vi "appEntry.vi"() -> ()   [LabVIEW 2018]
uses:
  type_sa_visit.ctl
  <vilib>/addons/database/Connection.llb/DB Tools Open Connec (String).vi
  <vilib>/addons/database/Connection.llb/Conn Execute.vi
  <vilib>/addons/database/Recordset.llb/Rec Fetch Recordset Data (R).vi
  <vilib>/addons/database/_DB Variant To Data/Database Variant To Data.xnode
  <vilib>/addons/database/NI_Database_API.lvlib
panel:
  in  "选项卡控件":enum32{"信息查询", "宿舍管理", "公寓管理", "系统管理"}(tab)
  in  "type_stu_apartment_visit":T1
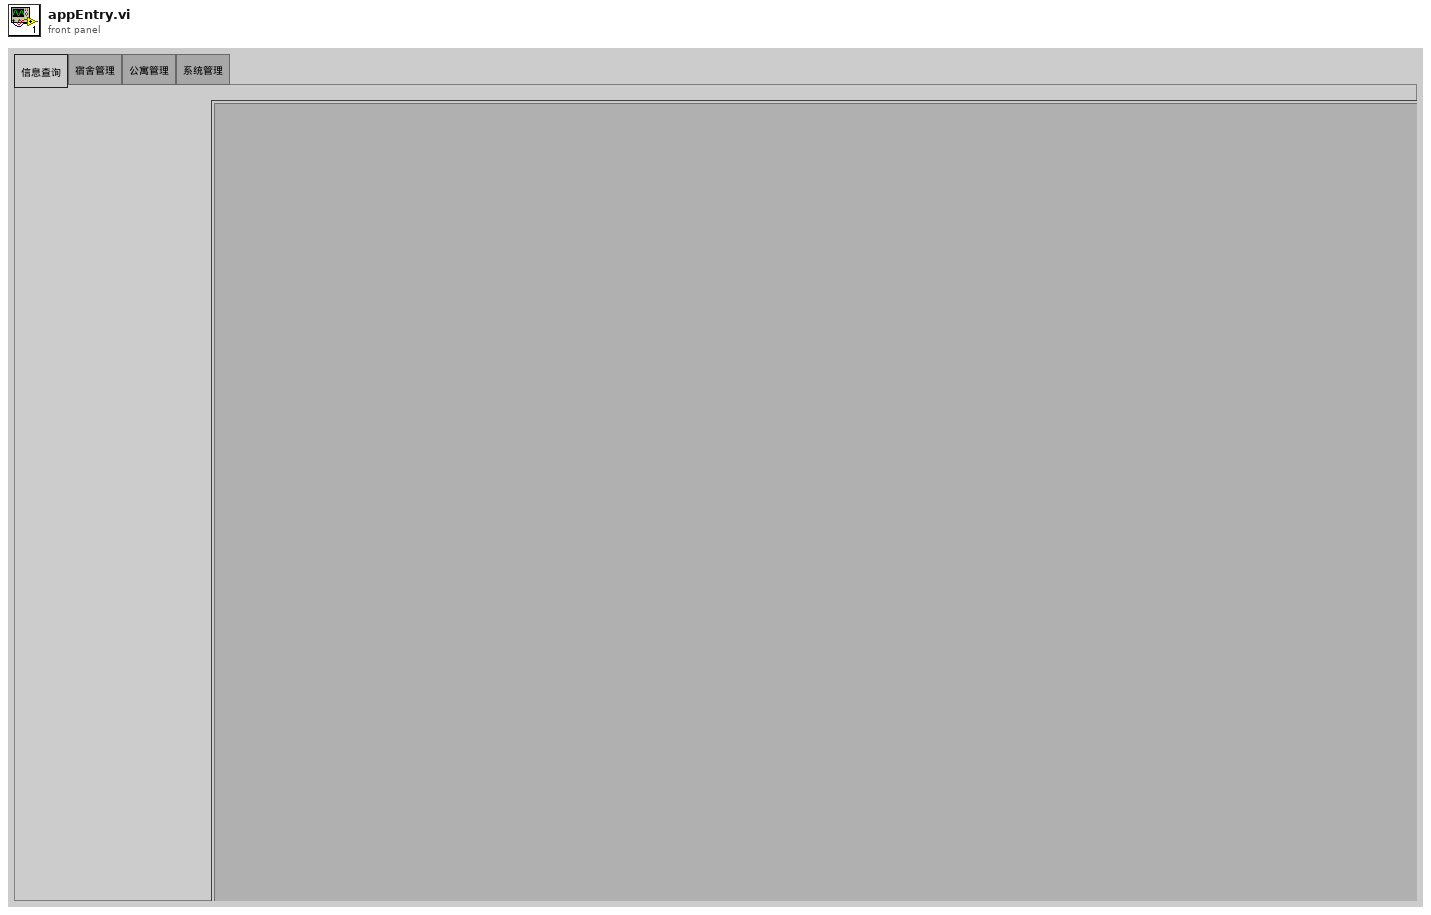
[diagram p1: front panel]
types:
  T1 = typedef "type_sa_visit.ctl" = cluster{"字符串":string, "字符串 2":string, "字符串 3":string, "字符串 4":string, "字符串 5":string, "字符串 6":string, "字符串 7":string, "字符串 8":string, "时间标识":timestamp, "时间标识 2":timestamp}
  T2 = typedef "NI_Database_API.lvlib/Conn ObjectReference.ctl" = refnum<k1>
  T3 = typedef "NI_Database_API.lvlib/Rec ObjectReference.ctl" = refnum<k1>
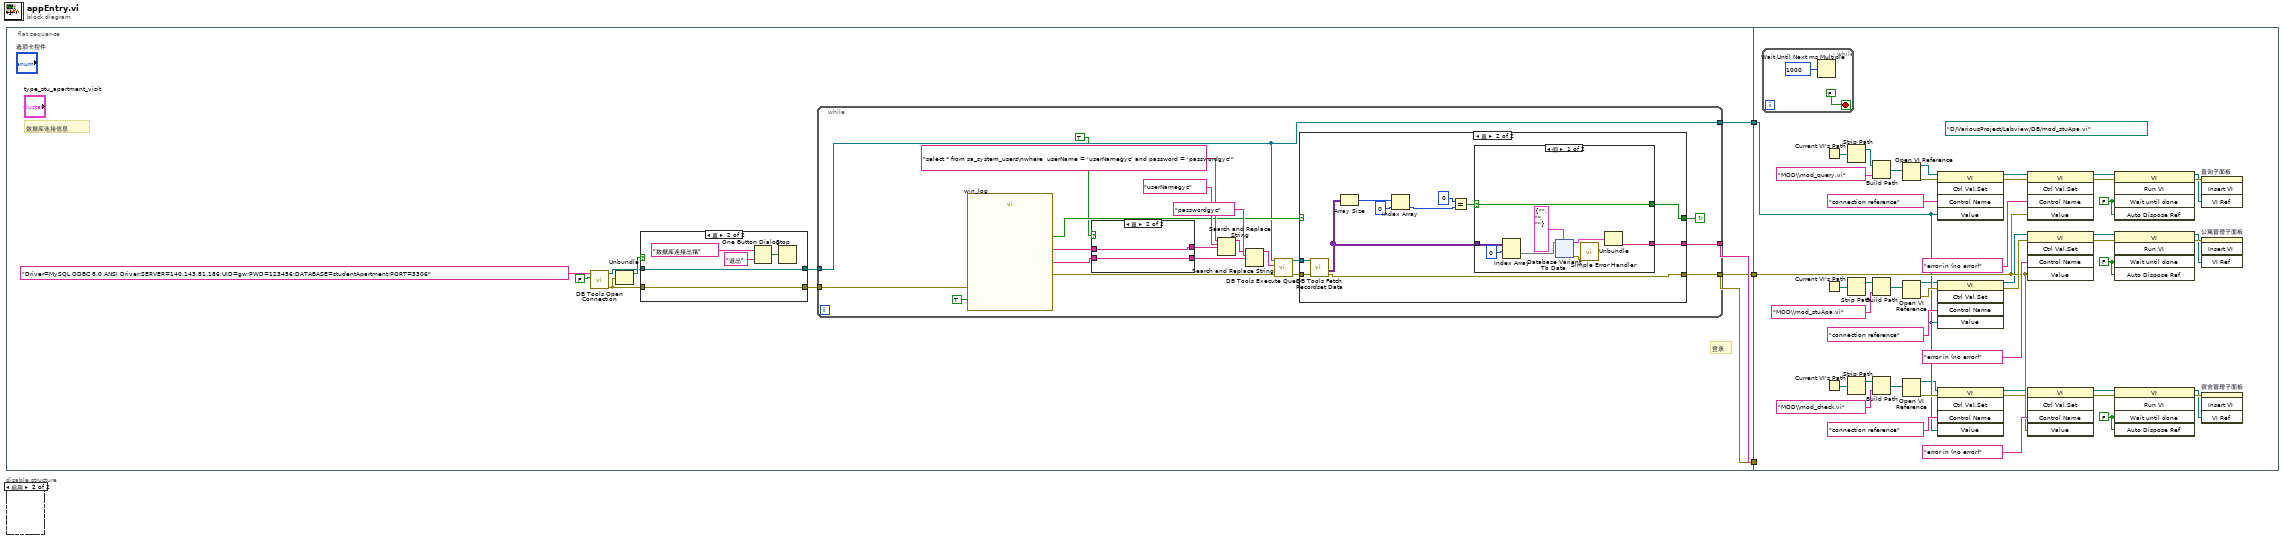
[diagram p0: block diagram]
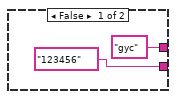
[diagram p3: hidden frame]
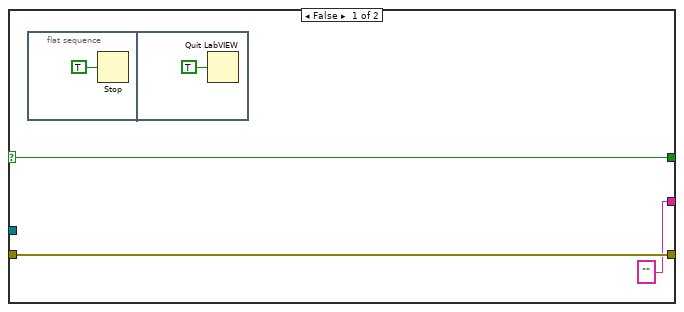
[diagram p4: hidden frame]
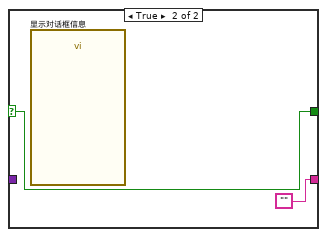
[diagram p5: hidden frame]
diagram:
  n1 = flat-sequence {
    tunnel: [w10] -> w4
    tunnel: [w9] -> w3
    tunnel: [w7] -> w2
    tunnel: [w7] -> w1
    tunnel: w4 -> [w193]
    tunnel: w3 -> [_]
    tunnel: w2 -> [_]
    tunnel: w1 -> [w195]
    frame #0 {
      # "登录"
      # "数据库连接信息"
      n2 = call-poly <vilib>:"DB Tools Open Connection.vi"("prompt? (F)"=FALSE, "connection information"="Driver=MySQL ODBC 8.0 ANSI Driver;SERVER=140.143.81.186;UID=gw;PWD=123456;DATABASE=studentApartment;PORT=3306") -> ("error out"=w12:errorcluster, "connection reference"=w13:T2)  [unwired: 6 in]
      n3 = Unbundle(w12) -> ("status"=w14:bool)  [unwired: 2 out]
      n4 = case shown="真" w14 {
        tunnel: w13 -> [w163 w166]
        tunnel: [w163 w166] -> w8
        tunnel: w12 -> [w162 w164]
        tunnel: [w162 w164] -> w11
        frame False {
        }
        frame True {
          n5 = One Button Dialog(message="数据库连接出错" ("消息"), button name ("OK")="退出" ("按钮名称（“确定”）")) -> (true=w167:bool)
          n6 = Stop(stop? (T)=w167) -> ()
        }
      }
      n7 = while {
        tunnel: w11 -> [w34]
        tunnel: w8 -> [w20]
        tunnel: [w26] -> w7
        tunnel: [w21] -> w9
        tunnel: [w20] -> w10
        stop <- w27 continue-if-true
        n8 = call "win_log.vi"("Enable"=TRUE, "error in (no error)"=w34) -> ("密码"=w17:string, "账号"=w18:string, "确定"=w28:bool, "error out"=w23:errorcluster)  [unwired: 14 in]
        n9 = case shown="真" TRUE {
          tunnel: w18 -> [_ w38]
          tunnel: w17 -> [_ w37]
          tunnel: ["gyc" w38] -> w16
          tunnel: ["123456" w37] -> w15
          frame False {
          }
          frame True {
          }
        }
        n10 = Search and Replace String(input string="select * from sa_system_users\nwhere  userName = 'userNamegyc' and password = 'passwordgyc'" ("SQL query"), search string="userNamegyc" ("搜索字符串"), replace string=w16) -> (result string=w29:string)  [unwired: 5 in, 3 out]
        n11 = Search and Replace String(input string=w29, search string="passwordgyc" ("搜索字符串"), replace string=w15) -> (result string=w22:string)  [unwired: 5 in, 3 out]
        n12 = call-poly <vilib>:"DB Tools Execute Query.vi"("error in (no error)"=w23, "SQL query"=w22, "connection reference"=w20) -> ("error out"=w24:errorcluster, "recordset reference"=w25:T3)  [unwired: 5 in]
        n13 = case shown="真" w28 {
          selector: w28 -> [w41 _]
          tunnel: w24 -> [w40 w46]
          tunnel: [w41 w49] -> w27
          tunnel: [w40 w48] -> w26
          tunnel: w25 -> [_ w47]
          tunnel: ["" w44] -> w21
          frame False {
            n14 = flat-sequence {
              frame #0 {
                n15 = Stop(stop? (T)=TRUE ("停止？(T)")) -> ()
              }
              frame #1 {
                n16 = Quit LabVIEW(quit? (T)=TRUE ("退出？(T)")) -> ()
              }
            }
          }
          frame True {
            n17 = call-poly <vilib>:"DB Tools Fetch Recordset Data.vi"("error in (no error)"=w46, "recordset reference"=w47) -> ("error out"=w48:errorcluster, "recordset data"=w45:variant[][])  [unwired: 3 in, 1 out]
            n18 = Array Size(array=w45) -> (size(s)=w54:i32[])
            n19 = Index Array(array=w54, index=0 ("索引")) -> (element=w52:i32)
            n20 = Equal?(x=0, y=w52) -> (x = y?=w50:bool)
            n21 = case shown="假" w50 {
              selector: w50 -> [w62 w161]
              tunnel: [w62 w161] -> w49
              tunnel: w45 -> [w56 _]
              tunnel: [w55 ""] -> w44
              frame False {
                n22 = Index Array(array=w56, index (row)=0 ("索引 (行)")) -> (element=w59:variant[])  [unwired: 1 in]
                n23 = xnode "Database Variant To Data"("database variant"=w59, "type"=cluster{string, string, string} {"", "", ""}) -> ("data"=w60:cluster{string, string, string}, "error out"=w61:errorcluster)  [unwired: 1 in]
                n24 = call <vilib>:"Simple Error Handler.vi"("error in (no error)"=w61) -> ()  [unwired: 4 in, 5 out]
                n25 = Unbundle(w60) -> (w55:string)  [unwired: 2 out]
              }
              frame True {
                n26 = call "显示对话框信息"() -> ()  [unwired: 10 in, 2 out]
              }
            }
          }
        }
      }
    }
    frame #1 {
      w182 = FALSE
      w197 = FALSE
      (unwired) path "D:/VariousProject/Labview/DB/mod_stuApa.vi" ("VI路径")
      w208 = FALSE
      n27 = while {
        stop <- FALSE stop-if-true
        n28 = Wait Until Next ms Multiple(millisecond multiple=u32 1000 ("毫秒倍数")) -> ()  [unwired: 1 out]
      }
      n29 = Current VI's Path() -> (path=w188:path)
      n30 = Current VI's Path() -> (path=w177:path)
      n31 = Current VI's Path() -> (path=w172:path)
      n32 = Strip Path(path=w188) -> (stripped path=w187:path)  [unwired: 1 out]
      n33 = Strip Path(path=w177) -> (stripped path=w176:path)  [unwired: 1 out]
      n34 = Strip Path(path=w172) -> (stripped path=w171:path)  [unwired: 1 out]
      n35 = Build Path(base path=w187, name or relative path="MOD\\mod_query.vi") -> (appended path=w185:path)
      n36 = Build Path(base path=w176, name or relative path="MOD\\mod_stuApa.vi") -> (appended path=w174:path)
      n37 = Build Path(base path=w171, name or relative path="MOD\\mod_check.vi") -> (appended path=w169:path)
      n38 = Open VI Reference(vi path=w185) -> (vi reference=w189:refnum<vi>, error out=w215:errorcluster)  [unwired: 5 in]
      n39 = Open VI Reference(vi path=w174) -> (vi reference=w190:refnum<vi>, error out=w203:errorcluster)  [unwired: 5 in]
      n40 = Open VI Reference(vi path=w169) -> (vi reference=w173:refnum<vi>, error out=w206:errorcluster)  [unwired: 5 in]
      n41 = invoke class="VI" method="Ctrl Val.Set"(reference=w189, error in=w215, "Control Name"="connection reference", "Value"=w193) -> (reference out=w212:refnum<vi>, error out=w211:errorcluster)  [unwired: 1 in, 3 out]
      n42 = invoke class="VI" method="Ctrl Val.Set"(reference=w190, error in=w203, "Control Name"="connection reference", "Value"=w193) -> (reference out=w194:refnum<vi>, error out=w200:errorcluster)  [unwired: 1 in, 3 out]
      n43 = invoke class="VI" method="Ctrl Val.Set"(reference=w173, error in=w206, "Control Name"="connection reference", "Value"=w193) -> (reference out=w184:refnum<vi>, error out=w183:errorcluster)  [unwired: 1 in, 3 out]
      n44 = invoke class="VI" method="Ctrl Val.Set"(reference=w212, error in=w211, "Control Name"="error in (no error)" ("控件名"), "Value"=w195) -> (reference out=w210:refnum<vi>, error out=w209:errorcluster)  [unwired: 1 in, 3 out]
      n45 = invoke class="VI" method="Ctrl Val.Set"(reference=w194, error in=w200, "Control Name"="error in (no error)" ("控件名"), "Value"=w195) -> (reference out=w199:refnum<vi>, error out=w198:errorcluster)  [unwired: 1 in, 3 out]
      n46 = invoke class="VI" method="Ctrl Val.Set"(reference=w184, error in=w183, "Control Name"="error in (no error)" ("控件名"), "Value"=w195) -> (reference out=w179:refnum<vi>, error out=w178:errorcluster)  [unwired: 1 in, 3 out]
      n47 = invoke class="VI" method="Run VI"(reference=w210, error in=w209, "Wait until done"=w208, "Auto Dispose Ref"=w208) -> (reference out=w191:refnum<vi>, error out=w207:errorcluster)  [unwired: 1 in, 3 out]
      n48 = invoke class="VI" method="Run VI"(reference=w199, error in=w198, "Wait until done"=w197, "Auto Dispose Ref"=w197) -> (reference out=w192:refnum<vi>, error out=w196:errorcluster)  [unwired: 1 in, 3 out]
      n49 = invoke class="VI" method="Run VI"(reference=w179, error in=w178, "Wait until done"=w182, "Auto Dispose Ref"=w182) -> (reference out=w180:refnum<vi>, error out=w181:errorcluster)  [unwired: 1 in, 3 out]
      n50 = invoke on="查询子面板" class="SubPnl" method="Insert VI"(error in=w207, "VI Ref"=w191) -> ()  [unwired: 2 in, 4 out]
      n51 = invoke on="公寓管理子面板" class="SubPnl" method="Insert VI"(error in=w196, "VI Ref"=w192) -> ()  [unwired: 2 in, 4 out]
      n52 = invoke on="宿舍管理子面板" class="SubPnl" method="Insert VI"(error in=w181, "VI Ref"=w180) -> ()  [unwired: 2 in, 4 out]
    }
  }
  n53 = disable-structure shown="启用" {
    frame Disabled {
    }
    frame Enabled {
    }
  }
